vi "MakePathCompatible.vi"(11 "path string":string) -> (3 "path":path)   [LabVIEW 2020, in "CICD.lvlib"]
doc: "Make path compatible with OS (i.e. replace '/' with '\\' for windows systems)."
uses:
  CICD.lvlib
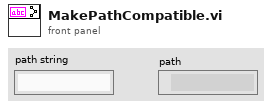
[diagram p1: front panel]
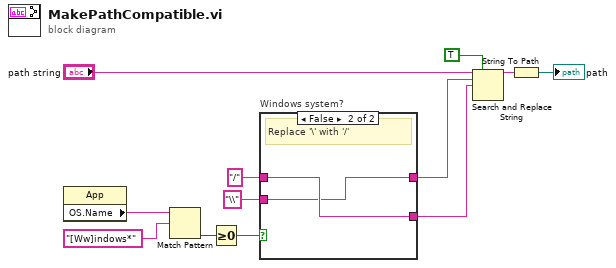
[diagram p0: block diagram]
diagram:
  n1 = property class="App"() -> ("OS.Name"=w8:string)  [unwired: 2 in, 2 out]
  n2 = Match Pattern(string=w8, regular expression="[Ww]indows*") -> (offset past match=w6:i32)  [unwired: 1 in, 3 out]
  n3 = Greater Or Equal To 0?(x=w6) -> (x >= 0?=w5:bool)
  n4 = case "Windows system?" shown="False" w5 {
    tunnel: [w14 w16] -> w4
    tunnel: [w13 w15] -> w3
    tunnel: "/" ("search string") -> [w13 w16]
    tunnel: "\\" ("search string") -> [w14 w15]
    frame True {
      # "Replace '/' with '\\'"
    }
    frame False {
      # "Replace '\\' with '/'"
    }
  }
  n5 = Search and Replace String(replace all?=TRUE ("replace all? (F)"), input string="path string", search string=w3, replace string=w4) -> (result string=w10:string)  [unwired: 4 in, 3 out]
  n6 = String To Path(string=w10) -> (path=→"path":path)
